vi "parse batch file (test).vi"() -> ()   [LabVIEW 2017]
uses:
  <vilib>/Utility/file.llb/Read Delimited Spreadsheet (string).vi
panel:
  out "Parsing errors":string
  out "all rows":string[][](array[string])
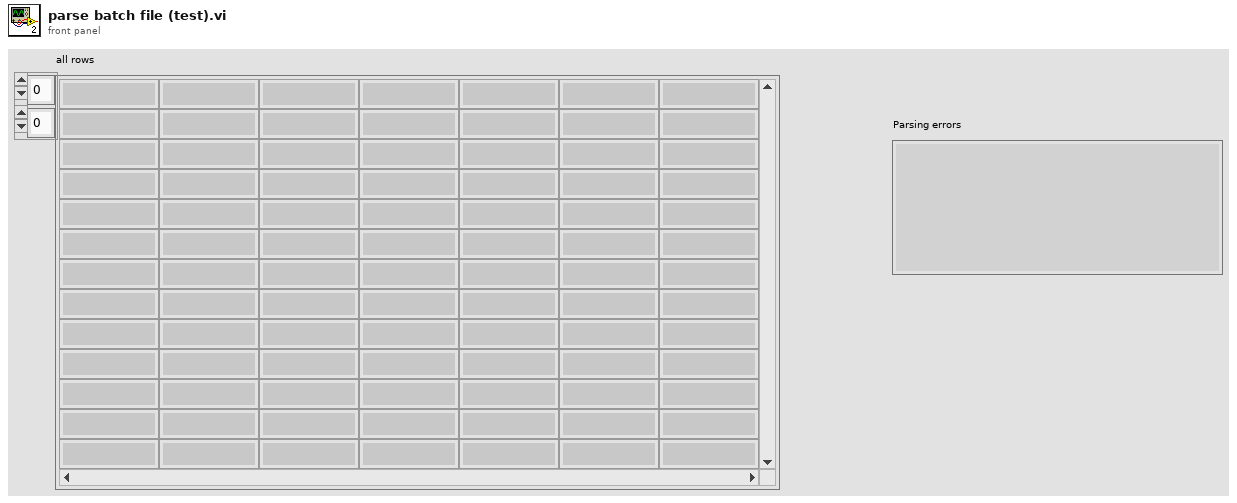
[diagram p1: front panel]
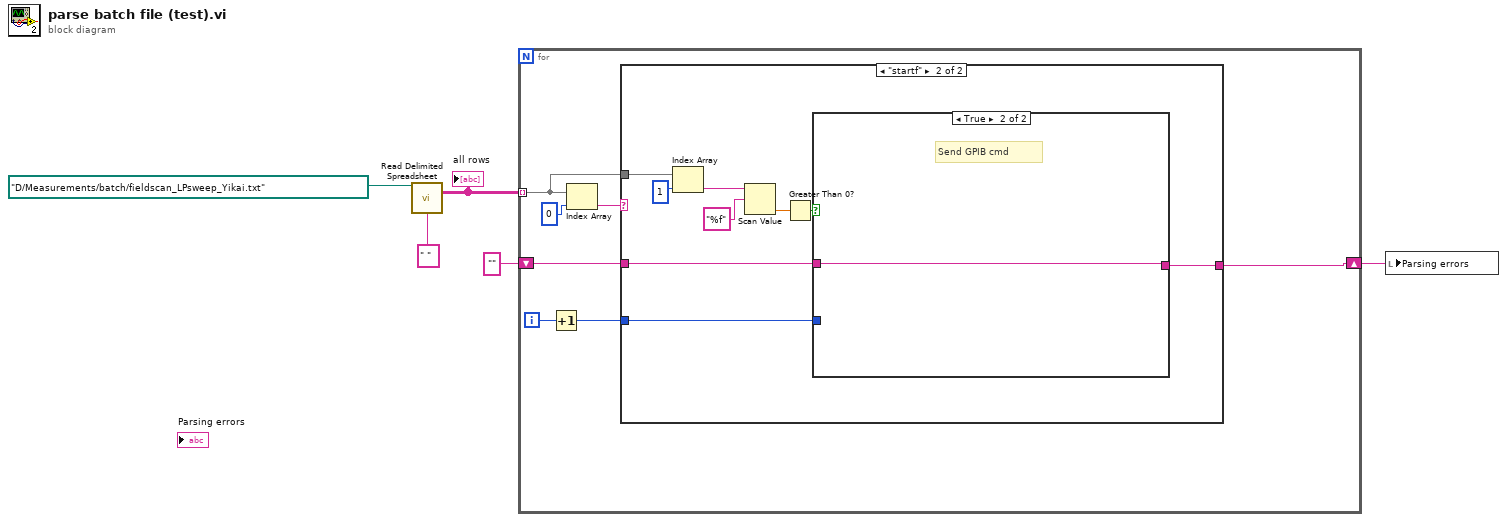
[diagram p0: block diagram]
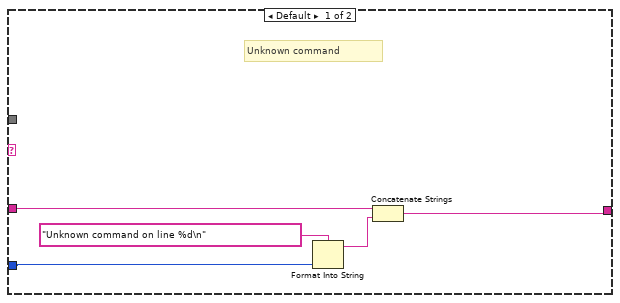
[diagram p2: hidden frame]
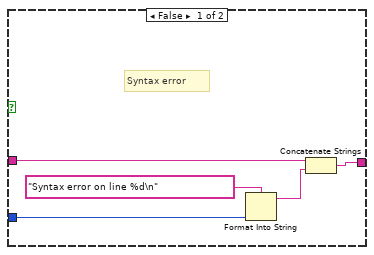
[diagram p3: hidden frame]
diagram:
  n1 = call-poly <vilib>:"Read Delimited Spreadsheet.vi"("file path (dialog if empty)"=path "D:/Measurements/batch/fieldscan_LPsweep_Yikai.txt", "delimiter (\\t)"=" " ("delimiter (\\t)")) -> ("all rows"=w3:string[][])  [unwired: 8 in, 5 out]
  "all rows" <- w3
  n2 = for {
    tunnel: w3 -> [w10] mode=indexing
    shift-right: [w6] -> w1
    shift-left: "" ("delimiter (\\t)") -> [w9]
    i -> [w8]
    n3 = Increment(x=w8) -> (x+1=w7:i32)
    n4 = Index Array(array=w10, index=0) -> (element=w11:string)
    n5 = case shown="\"startf\"" w11 {
      tunnel: w10 -> [_ w26]
      tunnel: w9 -> [w15 w20]
      tunnel: w7 -> [w13 w19]
      tunnel: [w14 w18] -> w6
      frame Default {
        # "Unknown command"
        n6 = Format Into String(format string="Unknown command on line %d\n" ("delimiter (\\t)"), w13) -> (resulting string=w17:string)  [unwired: 2 in, 1 out]
        n7 = Concatenate Strings(w15, w17) -> (w14:string)
      }
      frame "startf" {
        n8 = Index Array(array=w26, index=1) -> (element=w23:string)
        n9 = Scan Value(string=w23, format string="%f") -> (value=w22:dbl)  [unwired: 1 in, 1 out]
        n10 = Greater Than 0?(x=w22) -> (x > 0?=w21:bool)
        n11 = case shown="True" w21 {
          tunnel: w20 -> [w29 w32]
          tunnel: w19 -> [w30 _]
          tunnel: [w27 w32] -> w18
          frame False {
            # "Syntax error"
            n12 = Format Into String(format string="Syntax error on line %d\n" ("delimiter (\\t)"), w30) -> (resulting string=w28:string)  [unwired: 2 in, 1 out]
            n13 = Concatenate Strings(w29, w28) -> (w27:string)
          }
          frame True {
            # "Send GPIB cmd"
          }
        }
      }
    }
  }
  n14 = local write "Parsing errors"(w1) -> ()
